vi "DO-handler.vi"(9 "Output Control":T1, 11 "Current Output State":T1) -> (0 "output state changed":bool, 1 "hex integer string":string, 3 "DO Output":T1, 4 "number":u32, 6 "array":bool[](array[boolean]))   [LabVIEW 2020]
uses:
  controls/digital-output-cluster.ctl
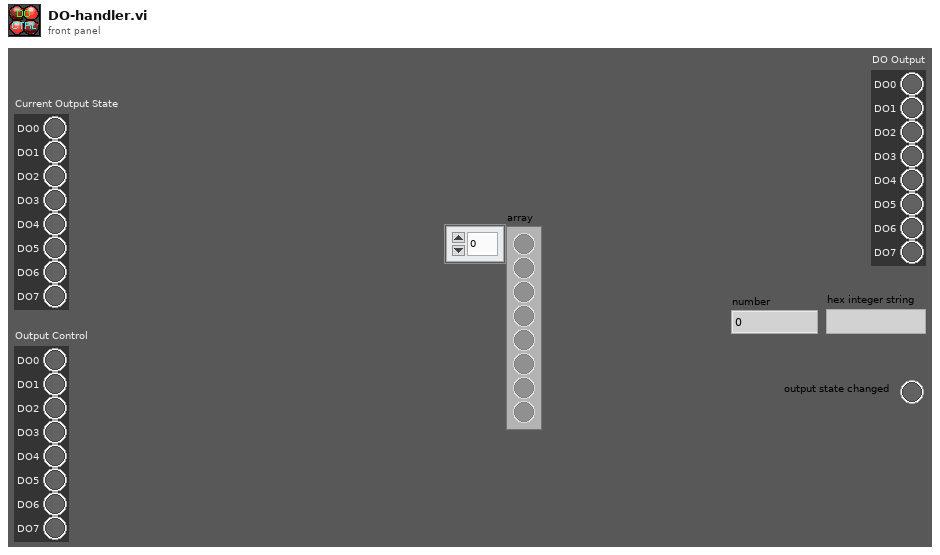
[diagram p1: front panel]
types:
  T1 = typedef "digital-output-cluster.ctl" = cluster{"DO0":bool, "DO1":bool, "DO2":bool, "DO3":bool, "DO4":bool, "DO5":bool, "DO6":bool, "DO7":bool}
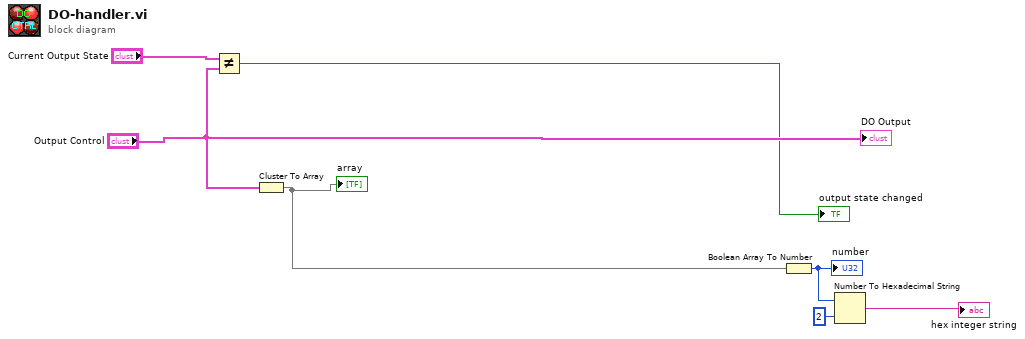
[diagram p0: block diagram]
diagram:
  n1 = Not Equal?(x="Current Output State", y="Output Control") -> (x != y?=→"output state changed":bool)
  n2 = Cluster To Array(cluster="Output Control") -> (array=w7:bool[])
  "array" <- w7
  n3 = Boolean Array To Number(Boolean array=w7) -> (number=w4:u32)
  "number" <- w4
  n4 = Number To Hexadecimal String(1:i16 2 ("width (-)"), 2:w4) -> (0:→"hex integer string":string)
  "DO Output" <- "Output Control"
